vi "DDE Server Example.vi"() -> ()   [LabVIEW 2015]
panel:
  in  "stop":bool
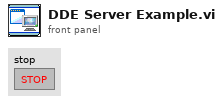
[diagram p1: front panel]
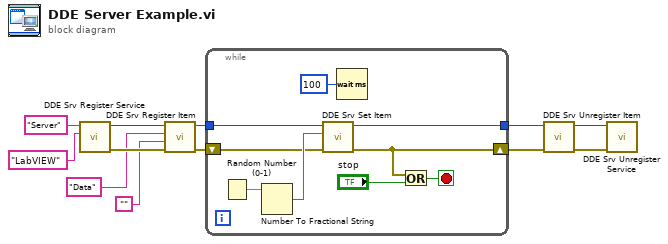
[diagram p0: block diagram]
diagram:
  n1 = call "DDE Srv Register Service.vi"("topic"="LabVIEW", "service"="Server") -> ("error out"=w9:errorcluster, "service refnum"=w10:u32)  [unwired: 6 in]
  n2 = call "DDE Srv Register Item.vi"("error in (no error)"=w9, "value"="", "item"="Data", "service refnum"=w10) -> ("error out"=w5:errorcluster, "item refnum"=w6:u32)  [unwired: 4 in]
  n3 = while {
    tunnel: w6 -> [w21]
    shift-right: [w16] -> w3
    shift-left: w5 -> [w17]
    tunnel: [w13] -> w4
    stop <- w14 stop-if-true
    n4 = Random Number (0-1)() -> (number: 0 to 1=w20:dbl)
    n5 = Number To Fractional String(number=w20) -> (F-format string=w19:string)  [unwired: 3 in]
    n6 = call "DDE Srv Set Item.vi"("error in (no error)"=w17, "value"=w19, "item refnum in"=w21) -> ("error out"=w16:errorcluster, "item refnum out"=w13:u32)  [unwired: 5 in]
    n7 = Wait (ms)(milliseconds to wait=u32 100) -> ()  [unwired: 1 out]
    n8 = Or(x=w16, y="stop") -> (x .or. y?=w14:bool)
  }
  n9 = call "DDE Srv Unregister Item.vi"("error in (no error)"=w3, "item refnum"=w4) -> ("error out"=w1:errorcluster, "service refnum"=w2:u32)  [unwired: 6 in]
  n10 = call "DDE Srv Unregister Service.vi"("error in (no error)"=w1, "service refnum"=w2) -> ()  [unwired: 7 in, 1 out]
